vi "4_Virtual_Channels.vi"(8 "error in (no error)":errorcluster) -> (0 "error out":errorcluster)   [LabVIEW 2014]
uses:
  SwabianInstruments.TimeTagger
panel:
  out "delay, ps":i64
  out "getData":dbl[](array[numeric]) format="%#.2f"
  # "Here, we have used a coincidence window that coincides just with the propagation delay\nbetween ch 1 and ch 2. Due to jitter, approximately half of the coincidence counts\nfall outside of this coincidence range. Therefore the coincidence countrate is\napproximately half of the original count rate."
  # "Measured propagation delay between channels 1 and 2"
  # "Measured count rates, counts/s"
  # "channel 1"
  # "channel 2"
  # "coincidences"
  # "combined channel 1 and channel 2"
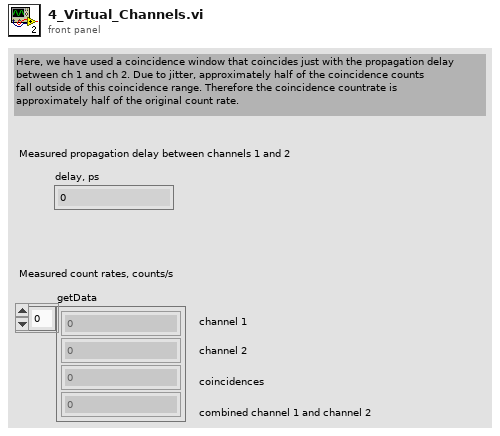
[diagram p1: front panel]
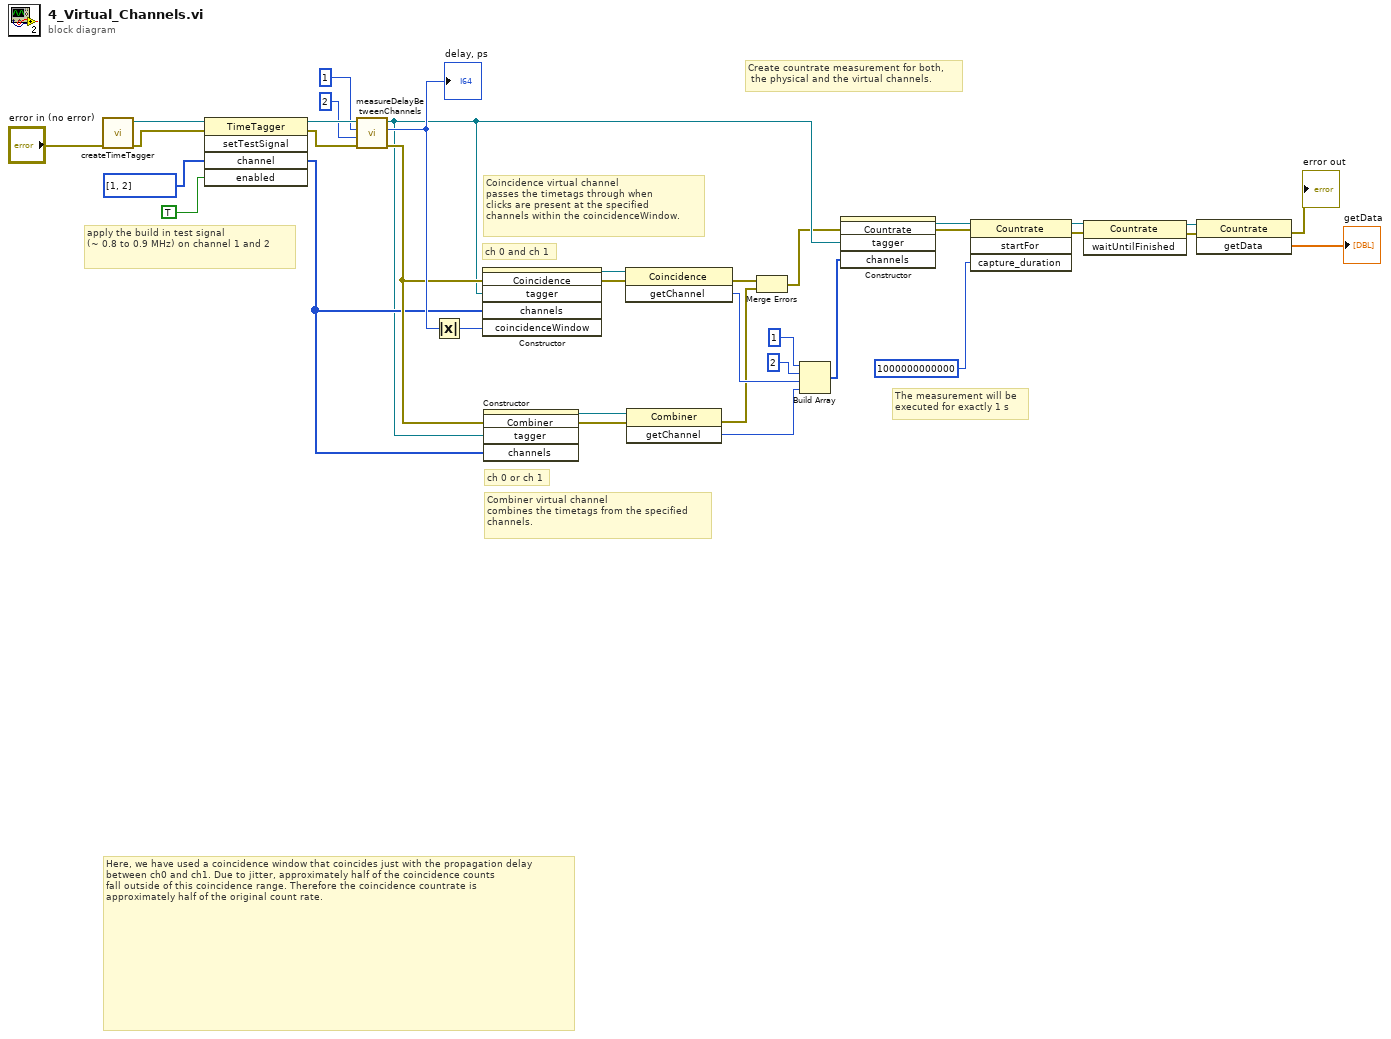
[diagram p0: block diagram]
diagram:
  # "The measurement will be\nexecuted for exactly 1 s"
  # "Create countrate measurement for both,\n the physical and the virtual channels."
  # "Combiner virtual channel\ncombines the timetags from the specified \nchannels."
  # "Coincidence virtual channel\npasses the timetags through when\nclicks are present at the specified \nchannels within the coincidenceWindow."
  # "ch 0 and ch 1"
  # "ch 0 or ch 1"
  # "Here, we have used a coincidence window that coincides just with the propagation delay\nbetween ch0 and ch1. Due to jitter, approximately half of the coincidence counts\nfall outside of this coincidence range. Therefore the coincidence countrate is\napproximately half of the original count rate."
  # "apply the build in test signal\n(~ 0.8 to 0.9 MHz) on channel 1 and 2"
  n1 = call "createTimeTagger.vi"("error in (no error)"="error in (no error)") -> ("error out"=w11:errorcluster, "TimeTagger ref out"=w12:refnum<k24>)  [unwired: 9 in]
  n2 = invoke class="TimeTagger" method="setTestSignal"(reference=w12, error in=w11, "channel"=i32[] [1, 2], "enabled"=TRUE) -> (reference out=w21:refnum<k24>, error out=w25:errorcluster, "channel"=w19:i32[])  [unwired: 1 in, 2 out]
  n3 = call "measureDelayBetweenChannels.vi"("error in (no error)"=w25, "channel_2"=2, "channel_1"=1, "TimeTagger ref in"=w21) -> ("error out"=w20:errorcluster, "measured delay, ps"=w22:i64, "TimeTagger ref out"=w16:refnum<k24>)  [unwired: 5 in]
  "delay, ps" <- w22
  n4 = Absolute Value(x=w22) -> (abs(x)=w27:i64)
  n5 = constructor class="Coincidence"(error in=w20, "tagger"=w16, "channels"=w19, "coincidenceWindow"=w27) -> (reference out=w32:refnum<k24>, error out=w31:errorcluster)  [unwired: 2 in, 4 out]
  n6 = constructor class="Combiner"(error in=w20, "tagger"=w16, "channels"=w19) -> (reference out=w34:refnum<k24>, error out=w33:errorcluster)  [unwired: 2 in, 3 out]
  n7 = invoke class="Coincidence" method="getChannel"(reference=w32, error in=w31) -> (error out=w15:errorcluster, "getChannel"=w24:i32)  [unwired: 1 in, 1 out]
  n8 = invoke class="Combiner" method="getChannel"(reference=w34, error in=w33) -> (error out=w14:errorcluster, "getChannel"=w23:i32)  [unwired: 1 in, 1 out]
  n9 = Merge Errors(w15, w14) -> (w13:errorcluster)
  n10 = Build Array(1 ("element"), 2 ("element"), w24, w23) -> (w30:i32[])
  n11 = constructor class="Countrate"(error in=w13, "tagger"=w16, "channels"=w30) -> (reference out=w7:refnum<k24>, error out=w8:errorcluster)  [unwired: 2 in, 3 out]
  n12 = invoke class="Countrate" method="startFor"(reference=w7, error in=w8, "capture_duration"=i64 1000000000000) -> (reference out=w6:refnum<k24>, error out=w5:errorcluster)  [unwired: 1 in, 2 out]
  n13 = invoke class="Countrate" method="waitUntilFinished"(reference=w6, error in=w5) -> (reference out=w4:refnum<k24>, error out=w3:errorcluster)  [unwired: 1 in, 1 out]
  n14 = invoke class="Countrate" method="getData"(reference=w4, error in=w3) -> (error out=→"error out":errorcluster, "getData"=→"getData":dbl[])  [unwired: 1 in, 1 out]
